vi "Get Clear Image.vi"(8 "error in (no error)":errorcluster) -> (0 "error out":errorcluster, 2 "Picture":picture)   [LabVIEW 2016, in "VI Reference Control.lvclass"]
uses:
  VI Reference Control.lvclass
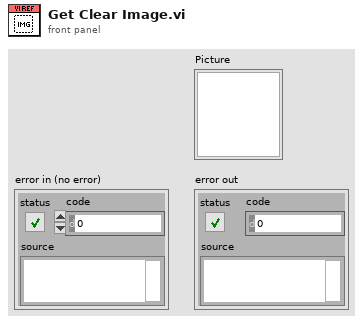
[diagram p1: front panel]
types:
  T1 = typedef "imagedata.ctl" = cluster{"image type":i32, "image depth":i32, "image":u8[], "mask":u8[], "colors":u32[], "Rectangle":cluster{"left":i16, "top":i16, "right":i16, "bottom":i16}}
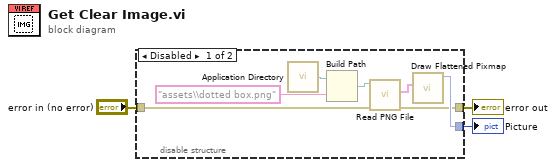
[diagram p0: block diagram]
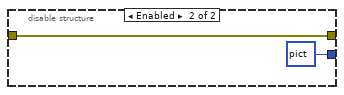
[diagram p2: hidden frame]
diagram:
  n1 = disable-structure shown="Disabled" {
    disable-tunnel: [w6 picture bytes[3390] ("Source Picture")] -> w1
    disable-tunnel: "error in (no error)" -> [w5 w11]
    disable-tunnel: [w4 w11] -> w2
    frame Disabled {
      n2 = call <vilib>:"Application Directory.vi"() -> ("Application Directory"=w10:path)
      n3 = Build Path(base path=w10, name or relative path="assets\\dotted box.png") -> (appended path=w8:path)
      n4 = call <vilib>:"Read PNG File.vi"("error in (no error)"=w5, "path to PNG file"=w8) -> ("error out"=w4:errorcluster, "image data"=w7:T1)  [unwired: 7 in, 1 out]
      n5 = call <vilib>:"Draw Flattened Pixmap.vi"("image data"=w7) -> ("new picture"=w6:picture)  [unwired: 8 in]
    }
    frame Enabled {
    }
  }
  "error out" <- w2
  "Picture" <- w1
